vi "First Step.vi"(8 "error in (no error)":errorcluster, 11 "Varian Magnet Scan.lvclass in":refnum<class "Varian Magnet Scan.lvclass">) -> (0 "error out":errorcluster, 2 "Current Position":dbl, 3 "Varian Magnet Scan.lvclass out":refnum<class "Varian Magnet Scan.lvclass">)   [LabVIEW 2009, in "Varian Magnet Scan.lvclass"]
doc: "Goto step #0 - the first step. If desired, the scanner may do this in a different way than usual (i.e. by preparing to move a long distance, or reset to home position.)"
uses:
  Varian Magnet Scan.lvclass
  Scanner/Scanner.lvclass
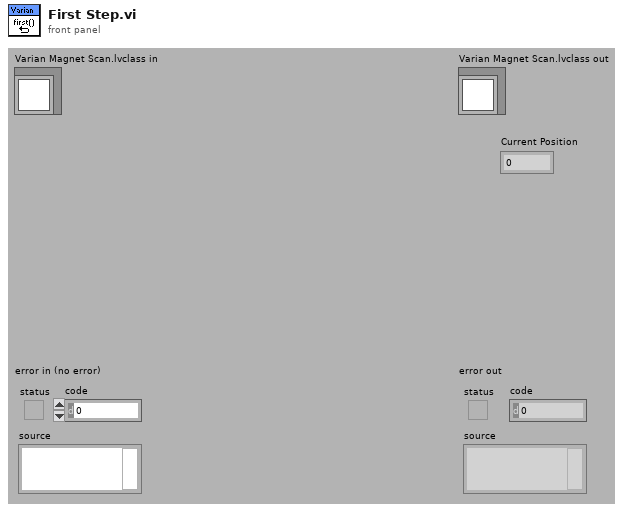
[diagram p1: front panel]
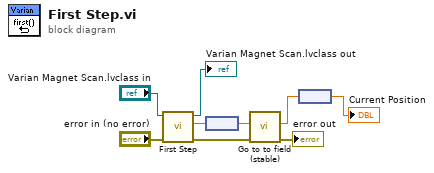
[diagram p0: block diagram]
diagram:
  n1 = call-parent "First Step.vi"("error in (no error)"="error in (no error)", "Scanner.lvclass in"="Varian Magnet Scan.lvclass in") -> ("error out"=w2:errorcluster, "Current Position"=w6:dbl, "Scanner.lvclass out"=→"Varian Magnet Scan.lvclass out":refnum<class "Varian Magnet Scan.lvclass">)  [unwired: 7 out]
  n2 = node(w6) -> (w5:dbl[unit])
  n3 = call "Go to to field (stable).vi"("error in"=w2, "Desired field"=w5) -> ("error out"=→"error out":errorcluster, "Current field"=w4:dbl[unit])  [unwired: 8 out]
  n4 = node(w4) -> (→"Current Position":dbl)
